vi "写入type.vi"(8 "error in (no error)":errorcluster caption="错误输入（无错误）", 10 "type":T1, 11 "data_combination输入":refnum<class "data_combination.lvclass">) -> (0 "error out":errorcluster caption="错误输出", 3 "data_combination输出":refnum<class "data_combination.lvclass">)   [LabVIEW 2016, in "潮位站数据传输.lvlib" / "data_combination.lvclass"]
uses:
  data_combination.lvclass
  data_combination.lvclass/data_combination.ctl
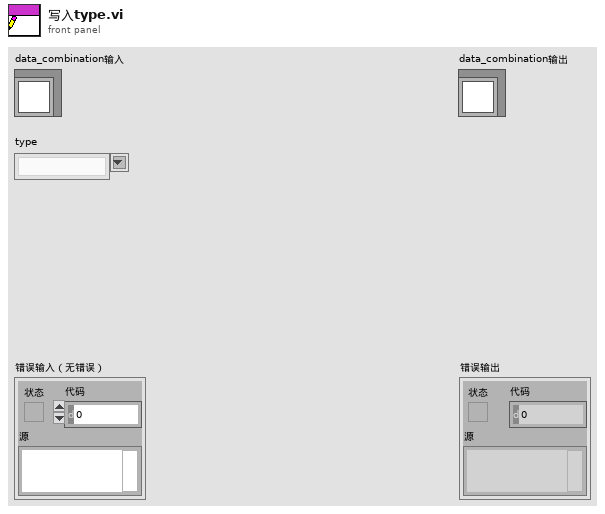
[diagram p1: front panel]
types:
  T1 = typedef "潮位站数据传输.lvlib/Type.ctl" = string
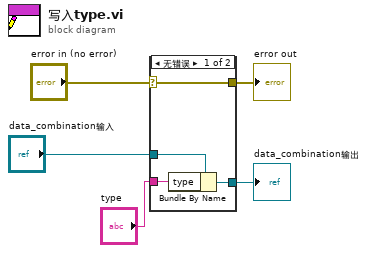
[diagram p0: block diagram]
diagram:
  n1 = case shown="无错误" "error in (no error)" {
    selector: "error in (no error)" -> [w9 w10]
    tunnel: [w9 w10] -> w4
    tunnel: [w7 w11] -> w2
    tunnel: "data_combination输入" -> [w8 w11]
    tunnel: "type" -> [w6 _]
    frame No Error {
      n2 = Bundle By Name(cluster=w8, "type"=w6) -> (w7:refnum<class "data_combination.lvclass">)
    }
    frame Error {
    }
  }
  "error out" <- w4
  "data_combination输出" <- w2
